vi "Array String(us) to Stamp.vi"(5 "time string(us)":string[](array[string])) -> (2 "time stamp(us)":timestamp[](array[timestamp]) format="%<%.6X\n%x>T")   [LabVIEW 2020]
panel:
  # "转换后有可能出现1us差"
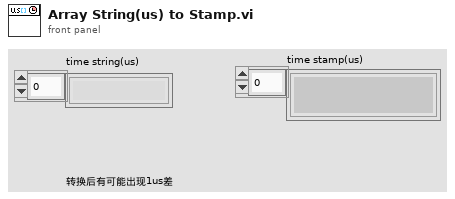
[diagram p1: front panel]
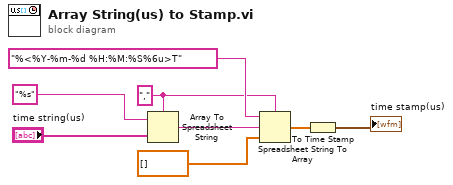
[diagram p0: block diagram]
diagram:
  w6 = "," ("delimiter (Tab)")
  n1 = Array To Spreadsheet String(delimiter (Tab)=w6, array="time string(us)", 3:"%s" ("format string")) -> (spreadsheet string=w5:string)
  n2 = Spreadsheet String To Array(delimiter (Tab)=w6, format string="%<%Y-%m-%d %H:%M:%S%6u>T", spreadsheet string=w5, array type (2D Dbl)=dbl[] []) -> (array=w3:dbl[])
  n3 = To Time Stamp(1:w3) -> (0:→"time stamp(us)":timestamp[])
